vi "Analogue Read.vi"(8 "error in":errorcluster, 11 "task/channels in":refnum<k21>) -> (0 "error out":errorcluster, 1 "RPM":i32[](array[knob]) scale=0.0..200.0, 2 "measured force":dbl[](array[numeric]), 3 "task out":refnum<k21>)   [LabVIEW 2021]
uses:
  <vilib>/Analysis/3filter.llb/Filter Passband Type.ctl
  <vilib>/DAQmx/read.llb/DAQmx Read (Analog 1D DBL NChan 1Samp).vi
  <vilib>/DAQmx/miscellaneous.llb/DAQmx Fill In Error Info.vi
  <vilib>/ptbypt/NI_PtbyPt.lvlib
  <vilib>/Analysis/NI_AALBase.lvlib
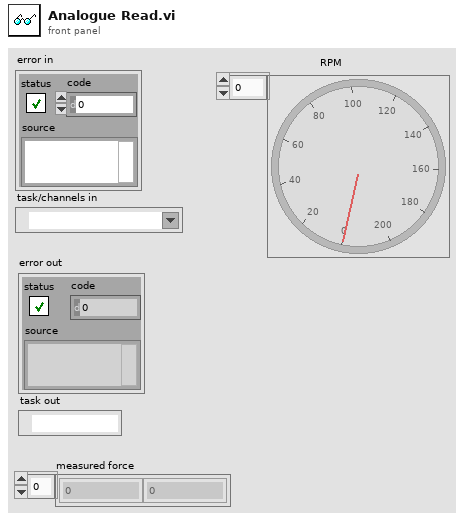
[diagram p1: front panel]
types:
  T1 = typedef "NI_AALBase.lvlib/Filter Passband Type.ctl" = enum32{"Lowpass", "Highpass", "Bandpass", "Bandstop"}
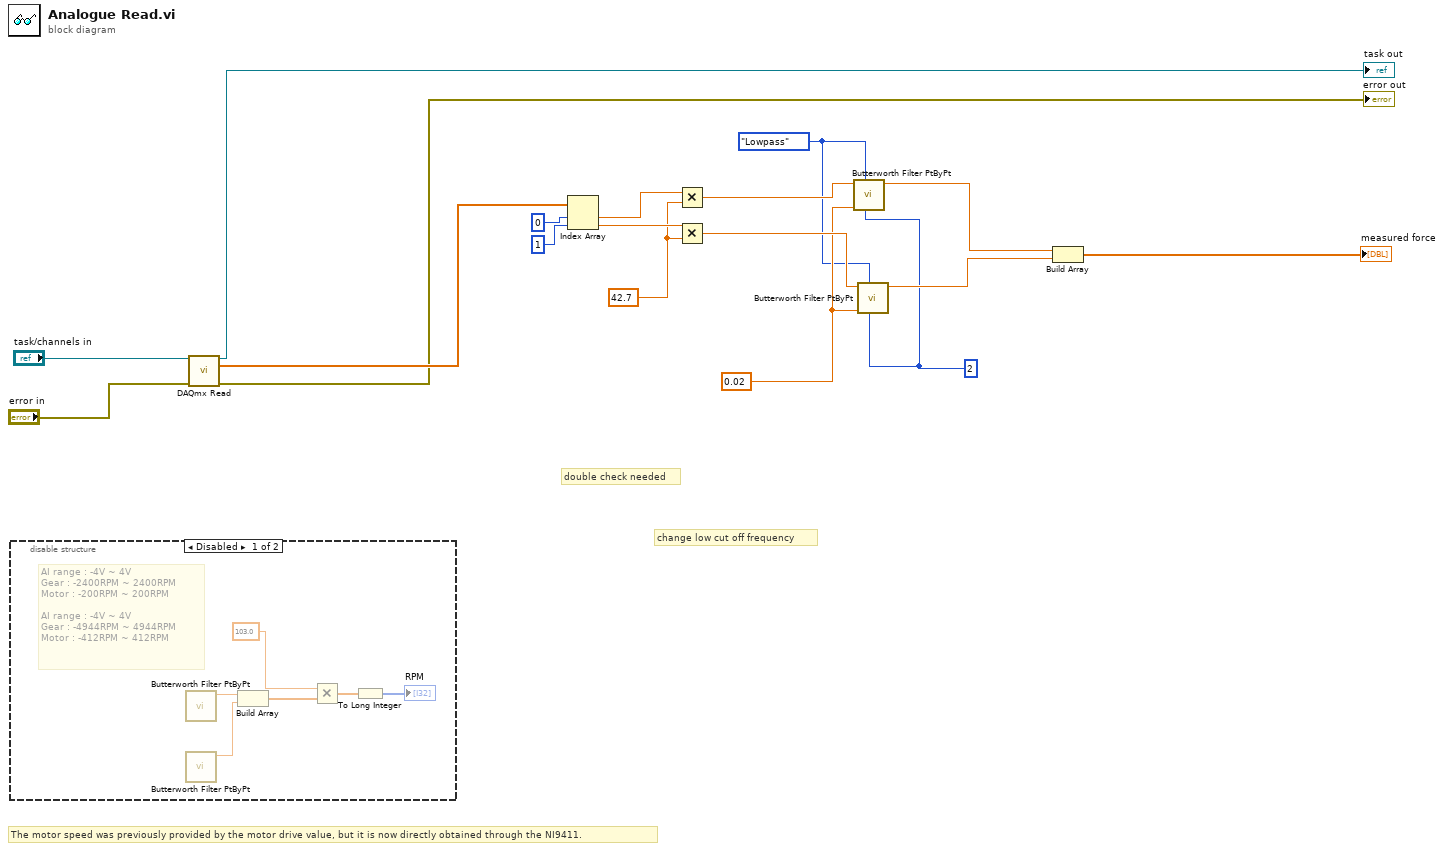
[diagram p0: block diagram]
diagram:
  w2 = 2 ("order")
  w4 = 0.02 ("low cutoff freq: fl")
  w1 = 42.7 ("y")
  w3 = Filter_Passband_Type."Lowpass" ("filter type")
  # "The motor speed was previously provided by the motor drive value, but it is now directly obtained through the NI9411."
  # "change low cut off frequency"
  # "double check needed"
  n1 = disable-structure shown="Disabled" {
    frame Disabled {
      # "AI range : -4V ~ 4V\nGear : -2400RPM ~ 2400RPM\nMotor : -200RPM ~ 200RPM\n\nAI range : -4V ~ 4V\nGear : -4944RPM ~ 4944RPM\nMotor : -412RPM ~ 412RPM"
      n2 = call <vilib>:"Butterworth Filter PtByPt.vi"() -> ("Filtered x"=w22:dbl)  [unwired: 9 in, 1 out]
      n3 = call <vilib>:"Butterworth Filter PtByPt.vi"() -> ("Filtered x"=w23:dbl)  [unwired: 9 in, 1 out]
      n4 = Build Array(w22, w23) -> (w24:dbl[])
      n5 = Multiply(x=103.0, y=w24) -> (x*y=w21:dbl[])
      n6 = To Long Integer(number=w21) -> (32bit integer=→"RPM":i32[])
    }
    frame Enabled {
    }
  }
  n7 = call-poly <vilib>:"DAQmx Read.vi"("task/channels in"="task/channels in", "error in"="error in") -> ("task out"=→"task out":refnum<k21>, "data"=w7:dbl[], "error out"=→"error out":errorcluster)  [unwired: 11 in]
  n8 = Index Array(array=w7, index #1=0 ("index"), index #2=1 ("index")) -> (element #1=w10:dbl, element #2=w9:dbl)
  n9 = Multiply(x=w10, y=w1) -> (x*y=w11:dbl)
  n10 = Multiply(x=w9, y=w1) -> (x*y=w8:dbl)
  n11 = call <vilib>:"Butterworth Filter PtByPt.vi"("order"=w2, "filter type"=w3, "low cutoff freq: fl"=w4, "x"=w11) -> ("Filtered x"=w16:dbl)  [unwired: 5 in, 1 out]
  n12 = call <vilib>:"Butterworth Filter PtByPt.vi"("order"=w2, "filter type"=w3, "low cutoff freq: fl"=w4, "x"=w8) -> ("Filtered x"=w15:dbl)  [unwired: 5 in, 1 out]
  n13 = Build Array(w16, w15) -> (→"measured force":dbl[])
